vi "Loop_ACT.vi"() -> ()   [LabVIEW 2017, in "Wing.lvlib"]
uses:
  Wing.lvlib
  _SHARE ALL/RoboRio Share All/SRX Share All/TypeDefs SRX/Cluster_SRX_Mode and Value.ctl
  System Drivers/Phoenix-LabVIEW/Motor Controller/Controls/CTRE_Phoenix_MotorControl_ControlMode.ctl
  _SHARE ALL/RoboRio Share All/SRX Share All/TypeDefs SRX/Cluster_SRX_Common Runtime Data.ctl
  _SHARE ALL/RoboRio Share All/SRX Share All/TypeDefs SRX/Cluster_SRX_Error Calculations.ctl
  _SHARE ALL/RoboRio Share All/SRX Share All/TypeDefs SRX/Cluster_SRX_Voltage Out Data.ctl
  _SHARE ALL/RoboRio Share All/SRX Share All/TypeDefs SRX/Cluster_SRX_Sensor Out Data.ctl
  _SHARE ALL/Global Share All/Global_STOP.vi
  Global_SM Write_Data Out.vi
  Global_ACT Write_Data Out.vi
panel:
  out "Common Runtime Data Out":T1 {"Temp" format="%.1f"; "Voltage"."Bus" format="%.3f"; "Voltage"."Output" format="%.3f"; "Voltage"."Percent" format="%.3f"; "Current" format="%.2f"}
  out "Mode And Value":T5 {"Mode" items=["PercentOutput"=0, "Position"=1, "Velocity"=2, "Current"=3, "Follower"=5, "MotionProfile"=6, "MotionMagic"=7, "MotionMagicArc"=8, "MotionProfileArc"=10, "Disabled"=15]}
  out "Cycle Time (S)":dbl format="%.3g"
  in  "Target Time(ms)":u32=50
  # "C"
  # "Units"
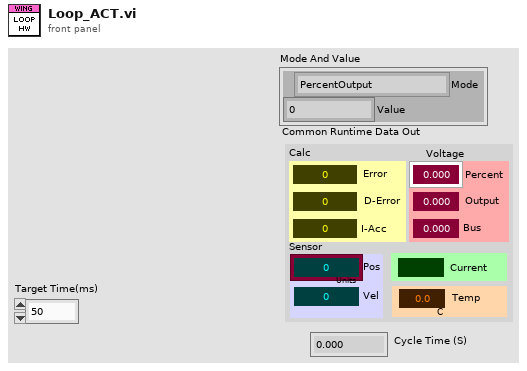
[diagram p1: front panel]
types:
  T1 = typedef "Cluster_SRX_Common Runtime Data.ctl" = cluster{"Calc":T2, "Voltage ":T3, "Sensor":T4, "Current":dbl, "Temp":dbl}
  T2 = typedef "Cluster_SRX_Error Calculations.ctl" = cluster{"Error":i32, "D-Error":dbl, "I-Acc":dbl}
  T3 = typedef "Cluster_SRX_Voltage Out Data.ctl" = cluster{"Percent":dbl, "Output":dbl, "Bus":dbl}
  T4 = typedef "Cluster_SRX_Sensor Out Data.ctl" = cluster{"Pos":i32, "Vel":i32}
  T5 = typedef "Cluster_SRX_Mode and Value.ctl" = cluster{"Mode":T6, "Value":dbl}
  T6 = typedef "CTRE_Phoenix_MotorControl_ControlMode.ctl" = u16
  T7 = typedef "WPI_MotorControlDeviceRef.ctl" = cluster{"DeviceStatus":errorcluster, "Type":T8, "PWM":cluster{"PWM Channel":T9, "DeadBand":T10}, "CAN":cluster{"Device Number":u8, "SetOutput VI Ref":variant, "GetOutput VI Ref":variant, "Enable VI Ref":variant, "Disable VI Ref":variant, "Data":variant}, "Invert":bool, "DIO PWM":cluster{"PWM \"Enable\" Channel":T9, "DIOChannel":T11, "PWM Rate":dbl}}
  T8 = typedef "WPI_MotorControlType.ctl" = enum16{"PWM", "CAN", "DIO PWM"}
  T9 = typedef "FPGA_DIOPWMChannel.ctl" = enum8{"PWM 0", "PWM 1", "PWM 2", "PWM 3", "PWM 4", "PWM 5", "PWM 6", "PWM 7", "PWM 8", "PWM 9", "PWM MXP 0", "PWM MXP 1", "PWM MXP 2", "PWM MXP 3", "PWM MXP 4", "PWM MXP 5", "PWM MXP 6", "PWM MXP 7", "PWM MXP 8", "PWM MXP 9", "Invalid"}
  T10 = typedef "WPI_PWMDeadband.ctl" = cluster{"Name":string, "maxPositivePwm":i32, "minPositivePwm":i32, "centerPwm":i32, "maxNegativePwm":i32, "minNegativePwm":i32, "angularRange":u16}
  T11 = typedef "FPGA_DIOChannel.ctl" = enum8{"DIO 0", "DIO 1", "DIO 2", "DIO 3", "DIO 4", "DIO 5", "DIO 6", "DIO 7", "DIO 8", "DIO 9", "DIO MXP 0", "DIO MXP 1", "DIO MXP 2", "DIO MXP 3", "DIO MXP 4", "DIO MXP 5", "DIO MXP 6", "DIO MXP 7", "DIO MXP 8", "DIO MXP 9", "DIO MXP 10", "DIO MXP 11", "DIO MXP 12", "DIO MXP 13", "DIO MXP 14", "DIO MXP 15", "SPI Port CS1", "SPI Port CS2", "SPI Port CS3", "SPI Port MISO", "SPI Port MOSI", "Invalid"}
  T12 = cluster{"CAN Talon SRX Ref":T7, " Actuator Output":dbl, "Actuator Input":dbl, "Target Time(ms)":u32, "Current Time":timestamp, "Previous Time":timestamp, "Cycle Time (S)":dbl, "Mode And Value":T5, "Common Runtime Data Out":T1}
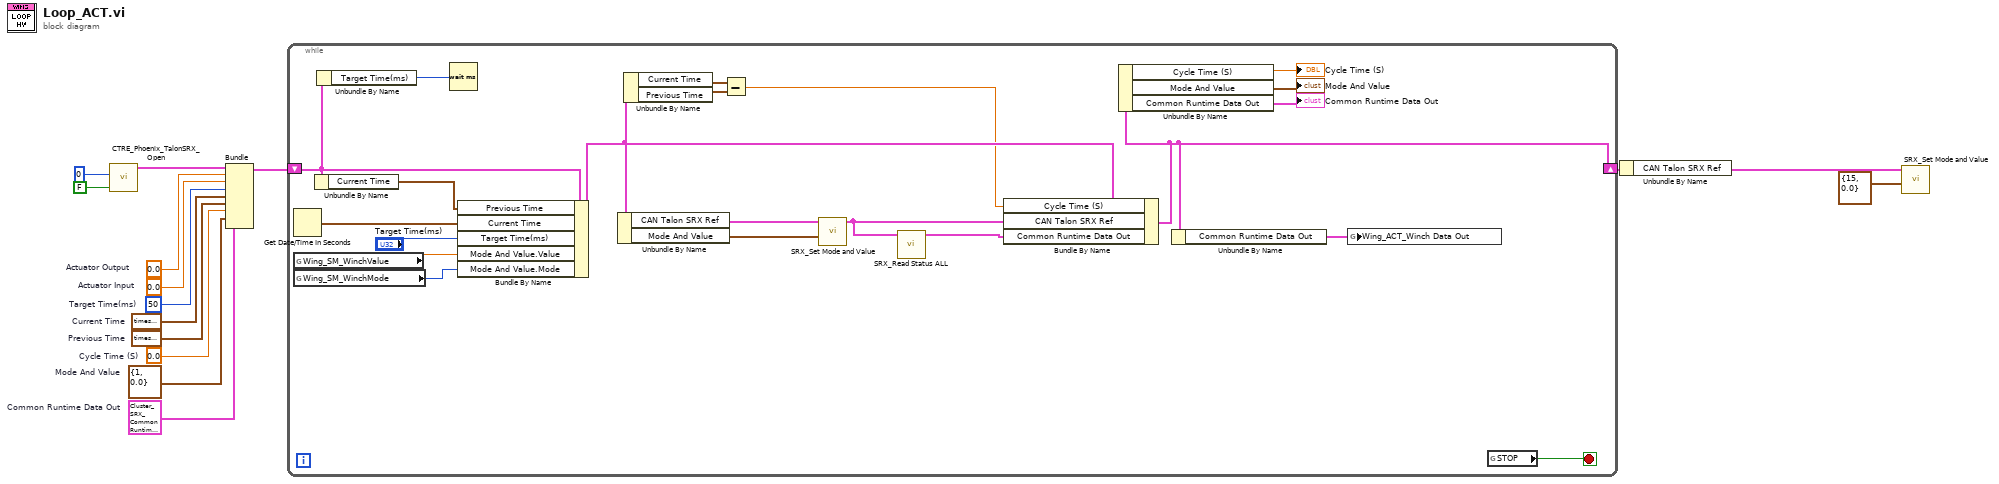
[diagram p0: block diagram]
diagram:
  w4 = T1 {"Calc"={"Error"=0, "D-Error"=0.0, "I-Acc"=0.0}, "Voltage "={"Percent"=0.0, "Output"=0.0, "Bus"=0.0}, "Sensor"={"Pos"=0, "Vel"=0}, "Current"=0.0, "Temp"=0.0}  # Common Runtime Data Out
  w5 = T5 {"Mode"=1, "Value"=0.0}  # Mode And Value
  w6 = 0.0  # Cycle Time (S)
  w15 = timestamp(0 s since 1904-01-01)  # Previous Time
  w14 = timestamp(0 s since 1904-01-01)  # Current Time
  w13 = u32 50  # Target Time(ms)
  w11 = 0.0  # Actuator Input
  w9 = 0.0  # Actuator Output
  n1 = call "CTRE_Phoenix_TalonSRX_Open.vi"("Invert"=FALSE, "Device Number"=u8 0) -> ("CAN Talon SRX Ref"=w8:T7)  [unwired: 8 in, 1 out]
  n2 = Bundle("CAN Talon SRX Ref"=w8, "Actuator Output"=w9, "Actuator Input"=w11, "Target Time(ms)"=w13, "Current Time"=w14, "Previous Time"=w15, "Cycle Time (S)"=w6, "Mode And Value"=w5, "Common Runtime Data Out"=w4) -> (w10:T12)  [unwired: 1 in]
  n3 = while {
    shift-right: [w25] -> w7
    shift-left: w10 -> [w27]
    stop <- w36 stop-if-true
    n4 = Get Date/Time In Seconds() -> (seconds since 1Jan1904=w33:timestamp)
    n5 = global read "Global_SM Write_Data Out.vi" "Wing_SM_WinchValue"() -> (w21:dbl)
    n6 = global read "Global_SM Write_Data Out.vi" "Wing_SM_WinchMode"() -> (w19:T6)
    n7 = Unbundle By Name(w27) -> ("Current Time"=w32:timestamp)
    n8 = Unbundle By Name(w27) -> ("Target Time(ms)"=w26:u32)
    n9 = Wait (ms)(milliseconds to wait=w26) -> ()  [unwired: 1 out]
    n10 = Bundle By Name(cluster=w27, "Previous Time"=w32, "Current Time"=w33, "Target Time(ms)"="Target Time(ms)", "Mode And Value.Value"=w21, "Mode And Value.Mode"=w19) -> (w28:T12)
    n11 = Unbundle By Name(w28) -> ("CAN Talon SRX Ref"=w35:T7, "Mode And Value"=w34:T5)
    n12 = Unbundle By Name(w28) -> ("Current Time"=w31:timestamp, "Previous Time"=w30:timestamp)
    n13 = Subtract(x=w31, y=w30) -> (x-y=w22:dbl)
    n14 = call "SRX_Set Mode and Value.vi"("Mode And Value"=w34, "PhoenixMotorControlDevRef"=w35) -> ("PhoenixMotorControlDevRef Out"=w20:T7)  [unwired: 8 in, 1 out]
    n15 = call "SRX_Read Status ALL.vi"("PhoenixMotorControlDevRef"=w20) -> ("Common Runtime Data Out"=w18:T1)  [unwired: 4 in, 6 out]
    n16 = Bundle By Name(cluster=w28, "Cycle Time (S)"=w22, "CAN Talon SRX Ref"=w20, "Common Runtime Data Out"=w18) -> (w25:T12)
    n17 = Unbundle By Name(w25) -> ("Cycle Time (S)"=→"Cycle Time (S)":dbl, "Mode And Value"=→"Mode And Value":T5, "Common Runtime Data Out"=→"Common Runtime Data Out":T1)
    n18 = Unbundle By Name(w25) -> ("Common Runtime Data Out"=w17:T1)
    n19 = global write "Global_ACT Write_Data Out.vi" "Wing_ACT_Winch Data Out"(w17) -> ()
    n20 = global read "Global_STOP.vi" "STOP"() -> (w36:bool)
  }
  n21 = Unbundle By Name(w7) -> ("CAN Talon SRX Ref"=w12:T7)
  n22 = call "SRX_Set Mode and Value.vi"("Mode And Value"=T5 {"Mode"=15, "Value"=0.0}, "PhoenixMotorControlDevRef"=w12) -> ()  [unwired: 8 in, 2 out]
